vi "Calc_Actuators_Elevation Control.vi"(0 "Elev_Setpoint":dbl format="%.1f", 3 "Vpot_Left":dbl=0.06 format="%.4f", 4 "Vpot_Right":dbl=0.14 format="%.4f") -> (17 "Power_Left":dbl format="%.4f", 18 "Power_Right":dbl format="%.4f")   [LabVIEW 2017]
uses:
  Type Definitions/typedef_cluster_Actuator Calibrations.ctl
panel:
  out "Wfm Chart":T1(graph)
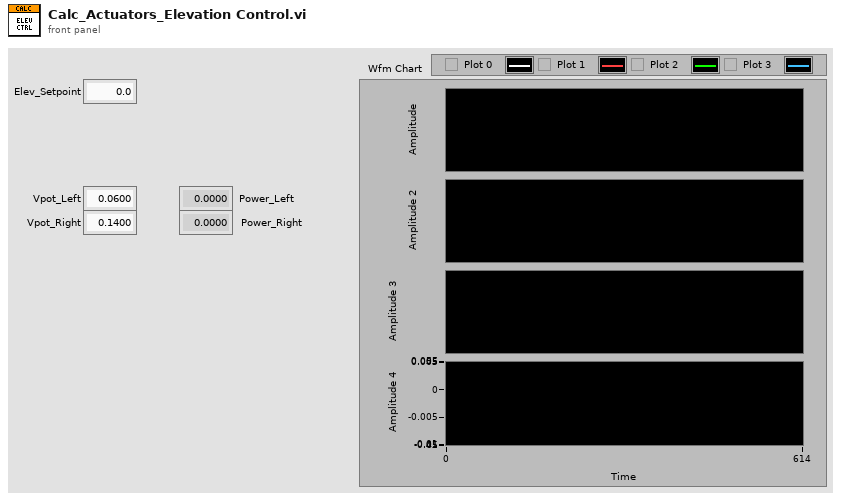
[diagram p1: front panel]
types:
  T1 = cluster{"Value":dbl, "Value":dbl, "Power OUT":dbl, "Power OUT":dbl}
  T2 = typedef "typedef_cluster_Actuator Calibrations.ctl" = cluster{"Vmax_Left":dbl, "Vmin_Left":dbl, "Vmax_Right":dbl, "Vmin_Right":dbl, "Elev_max":dbl, "Elev_min":dbl}
  T3 = cluster{"Value":dbl, "Value":dbl, "upper limit":dbl, "upper limit":dbl}
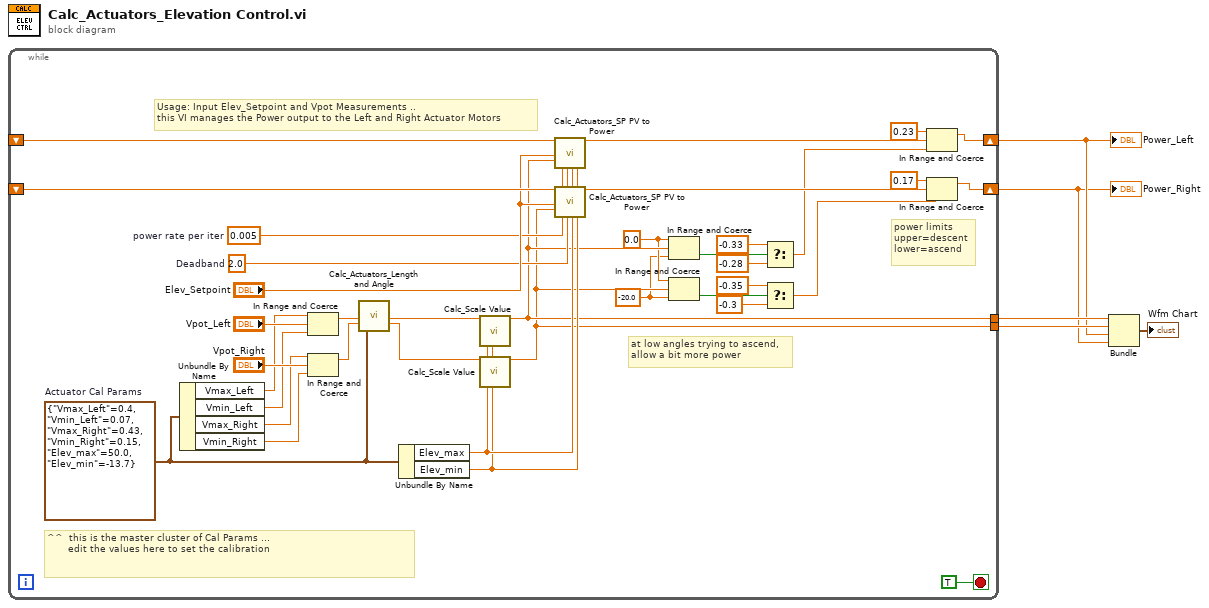
[diagram p0: block diagram]
diagram:
  n1 = while {
    shift-right: [w21] -> w3
    shift-left: _ -> [w33]
    shift-right: [w19] -> w2
    shift-left: _ -> [w32]
    tunnel: [w18] -> w5
    tunnel: [w17] -> w4
    stop <- TRUE stop-if-true
    w13 = -20.0 ("lower limit")
    w16 = 0.0 ("upper limit")
    w26 = 2.0  # Deadband
    w25 = 0.005  # power rate per iter
    w40 = T2 {"Vmax_Left"=0.4, "Vmin_Left"=0.07, "Vmax_Right"=0.43, "Vmin_Right"=0.15, "Elev_max"=50.0, "Elev_min"=-13.7}  # Actuator Cal Params
    # "at low angles trying to ascend,\nallow a bit more power"
    # "power limits\nupper=descent\nlower=ascend"
    # "^^  this is the master cluster of Cal Params ...\n       edit the values here to set the calibration"
    # "Usage: Input Elev_Setpoint and Vpot Measurements ..\nthis VI manages the Power output to the Left and Right Actuator Motors"
    n2 = Unbundle By Name(w40) -> ("Vmax_Left"=w37:dbl, "Vmin_Left"=w36:dbl, "Vmax_Right"=w35:dbl, "Vmin_Right"=w34:dbl)
    n3 = In Range and Coerce(upper limit=w37, x="Vpot_Left", lower limit=w36) -> (coerced(x)=w39:dbl)  [unwired: 1 out]
    n4 = In Range and Coerce(upper limit=w35, x="Vpot_Right", lower limit=w34) -> (coerced(x)=w38:dbl)  [unwired: 1 out]
    n5 = call "Calc_Actuators_Length and Angle.vi"("Vpot_Left"=w39, "Vpot_Right"=w38, "Actuator Cal Params"=w40) -> ("% Length_Left"=w30:dbl, "% Length_Right"=w31:dbl)  [unwired: 13 in, 2 out]
    n6 = Unbundle By Name(w40) -> ("Elev_max"=w29:dbl, "Elev_min"=w28:dbl)
    n7 = call "Calc_Scale Value.vi"("Normalized Value"=w30, "Max"=w29, "Min"=w28) -> ("Value"=w18:dbl)  [unwired: 16 in]
    n8 = call "Calc_Scale Value.vi"("Normalized Value"=w31, "Max"=w29, "Min"=w28) -> ("Value"=w17:dbl)  [unwired: 16 in]
    n9 = call "Calc_Actuators_SP PV to Power.vi"("Power IN"=w33, "Setpoint"="Elev_Setpoint", "Process Variable"=w18, "power rate per iter"=w25, "Deadband"=w26, "Limit Max"=w29, "Limit Min"=w28) -> ("Power OUT"=w22:dbl)  [unwired: 12 in]
    n10 = call "Calc_Actuators_SP PV to Power.vi"("Power IN"=w32, "Setpoint"="Elev_Setpoint", "Process Variable"=w17, "power rate per iter"=w25, "Deadband"=w26, "Limit Max"=w29, "Limit Min"=w28) -> ("Power OUT"=w20:dbl)  [unwired: 12 in]
    n11 = In Range and Coerce(upper limit=w16, x=w18, lower limit=w13) -> (In Range?=w15:bool)  [unwired: 1 out]
    n12 = In Range and Coerce(upper limit=w16, x=w17, lower limit=w13) -> (In Range?=w14:bool)  [unwired: 1 out]
    n13 = Select(t=-0.33, s=w15, f=-0.28 ("lower limit")) -> (s? t:f=w8:dbl)
    n14 = Select(t=-0.35, s=w14, f=-0.3 ("lower limit")) -> (s? t:f=w7:dbl)
    n15 = In Range and Coerce(upper limit=0.23, x=w22, lower limit=w8) -> (coerced(x)=w21:dbl)  [unwired: 1 out]
    n16 = In Range and Coerce(upper limit=0.17, x=w20, lower limit=w7) -> (coerced(x)=w19:dbl)  [unwired: 1 out]
  }
  "Power_Left" <- w3
  "Power_Right" <- w2
  n17 = Bundle("Value"=w5, "Value"=w4, "upper limit"=w3, "upper limit"=w2) -> (→"Wfm Chart":T3)  [unwired: 1 in]
